vi "subIsFileExist.vi"(1 "Path":path) -> (0 "isFileExist":bool)   [LabVIEW 2016]
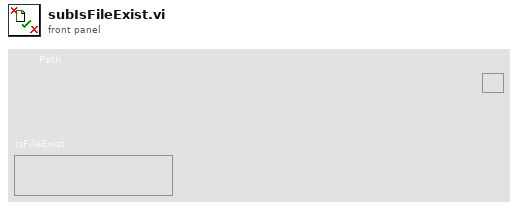
[diagram p1: front panel]
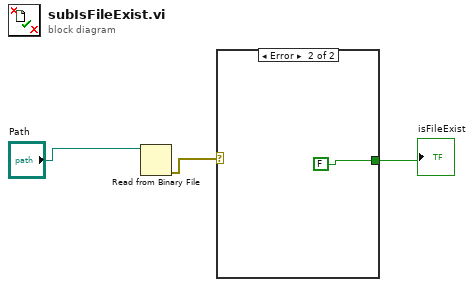
[diagram p0: block diagram]
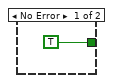
[diagram p2: hidden frame]
diagram:
  n1 = Read from Binary File(11:"Path") -> (0:w2:errorcluster)  [unwired: 5 in, 3 out]
  n2 = case shown="Error" w2 {
    tunnel: [TRUE FALSE] -> w1
    frame No Error {
    }
    frame Error {
    }
  }
  "isFileExist" <- w1
